vi "extracted dll error handler.vi"(8 "error in (no error)":errorcluster, 11 "error code":i32) -> (0 "error out":errorcluster)   [LabVIEW 2026, in "Nominal Core Streaming Engine.lvlib"]
uses:
  Nominal Core Streaming Engine.lvlib
  libnominalClient_64.dll
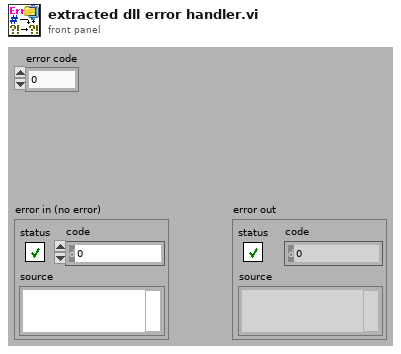
[diagram p1: front panel]
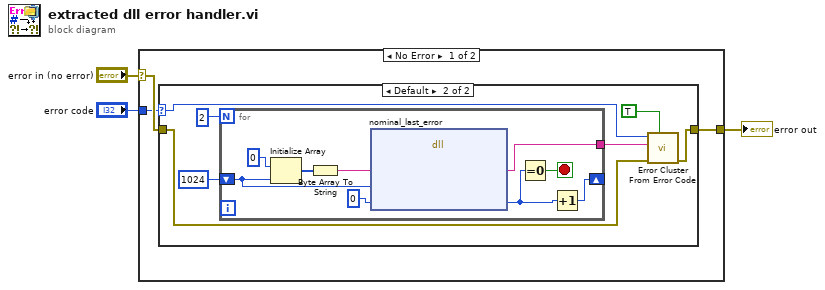
[diagram p0: block diagram]
diagram:
  n1 = case shown="No Error" "error in (no error)" {
    selector: "error in (no error)" -> [w6 w24]
    tunnel: [w4 w24] -> w2
    tunnel: "error code" -> [w5 _]
    frame No Error {
      n2 = case shown="Default" w5 {
        selector: w5 -> [_ w8]
        tunnel: w6 -> [w7 w14]
        tunnel: [w7 w13] -> w4
        frame 0 {
        }
        frame Default {
          n3 = for {
            N: 2 -> [_]
            tunnel: [w23] -> w11
            shift-right: [w20] -> _
            shift-left: 1024 -> [w18]
            stop <- w22 stop-if-true
            n4 = Initialize Array(u8 0, w18) -> (w15:u8[])
            n5 = Byte Array To String(unsigned byte array=w15) -> (string=w19:string)
            n6 = dll-call lib="C:/sw/ni-veristand-custom-device-nominal-core/source/libnominalClient_*.*" fn="nominal_last_error"("buf"=w19, "cap"=w18, "out_needed"=u32 0) -> ("buf"=w23:string, "out_needed"=w21:u32)  [unwired: 5 in, 2 out]
            n7 = Equal To 0?(x=w21) -> (x = 0?=w22:bool)
            n8 = Increment(x=w21) -> (x+1=w20:u32)
          }
          n9 = call <vilib>:"Error Cluster From Error Code.vi"("show call chain? (False)"=TRUE, "error in (no error)"=w14, "error message (\"\")"=w11, "error code (0)"=w8) -> ("error out"=w13:errorcluster)  [unwired: 5 in]
        }
      }
    }
    frame Error {
    }
  }
  "error out" <- w2
